vi "create shared data.vi"(8 "error in (no error)":errorcluster, 11 "Item Ref in":T1 format="%.0x") -> (0 "error out":errorcluster, 3 "Item Ref out":T1 format="%.0x")   [LabVIEW 2017, in "DSF System Explorer.lvlib"]
uses:
  DSF System Explorer.lvlib
  <vilib>/NI Veristand/Custom Device API/Custom Device Item Ref.ctl
  <vilib>/NI Veristand/Custom Device API/Custom Device API.lvlib
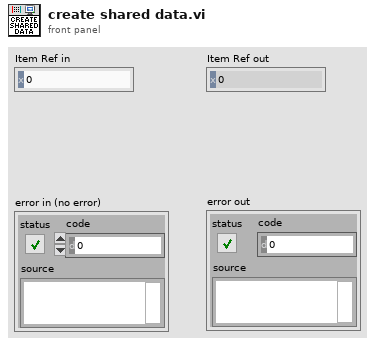
[diagram p1: front panel]
types:
  T1 = typedef "Custom Device API.lvlib/Custom Device Item Ref.ctl" = u64
  T2 = typedef "DSF System Explorer.lvlib/shared data ref.ctl" = refnum<data-value>
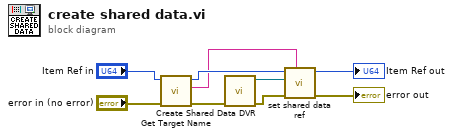
[diagram p0: block diagram]
diagram:
  n1 = call "Get Target Name.vi"("error in (no error)"="error in (no error)", "Node Ptr"="Item Ref in") -> ("error out"=w2:errorcluster, "target name"=w1:string, "Item Ref out"=w3:T1)  [unwired: 6 in, 1 out]
  n2 = call "Create Shared Data DVR.vi"("error in (no error)"=w2) -> ("error out"=w9:errorcluster, "Shared Data DVR"=w8:T2)  [unwired: 9 in]
  n3 = call "set shared data ref.vi"("target name"=w1, "error in (no error)"=w9, "shared data ref"=w8, "Node Ptr"=w3) -> ("error out"=→"error out":errorcluster, "Item Ref out"=→"Item Ref out":T1)  [unwired: 6 in]
